vi "On Drop.vi"(8 "error in (no error)":errorcluster, 10 "Actor in":refnum<class "Actor.lvclass">, 11 "Client Connection Handler Msg in":refnum<class "Server Connection Handler Msg.lvclass">) -> (0 "error out":errorcluster, 2 "Actor out":refnum<class "Actor.lvclass">, 3 "Client Connection Handler Msg out":refnum<class "Server Connection Handler Msg.lvclass">)   [LabVIEW 2021, in "Echo Reply Test With Server Manager.lvlib" / "Server Connection Handler Msg.lvclass"]
uses:
  Server Connection Handler Msg.lvclass
  <vilib>/ActorFramework/Actor/Actor.lvclass
  Server Connection Handler Msg.lvclass/Server Connection Handler Msg.ctl
  WS Test Server Subscriber/WS Test Server Subscriber.lvclass
  C:/Program Files/National Instruments/LabVIEW 2021/vi.lib/ActorFramework/Actor/Actor.lvclass
  C:/Projects/WebSocket-Actor/Examples/Echo Reply Test With Server Manager/WS Test Server Subscriber/WS Test Server Subscriber.lvclass
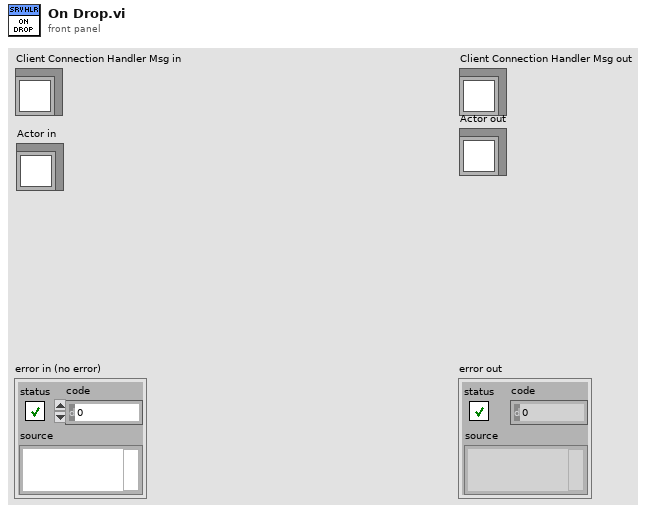
[diagram p1: front panel]
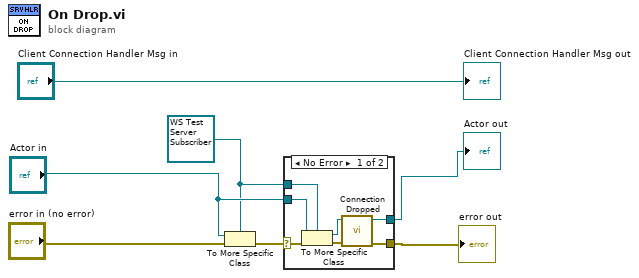
[diagram p0: block diagram]
diagram:
  w2 = refnum<class "WS Test Server Subscriber.lvclass"> refnum ("Echo Reply Test With Server Manager.lvlib:WS Test Server Subscriber.lvclass")
  n1 = To More Specific Class(target class=w2, reference="Actor in", error in="error in (no error)") -> (error out=w7:errorcluster)  [unwired: 1 out]
  n2 = case shown="No Error" w7 {
    selector: w7 -> [w13 w15]
    tunnel: [w14 w15] -> w5
    tunnel: w2 -> [w11 w16]
    tunnel: "Actor in" -> [w10 _]
    tunnel: [w8 w16] -> w3
    frame No Error {
      n3 = To More Specific Class(target class=w11, reference=w10, error in=w13) -> (specific class reference=w9:refnum<class "WS Test Server Subscriber.lvclass">, error out=w12:errorcluster)
      n4 = call "Connection Dropped.vi"("error in (no error)"=w12, "WS Test Server Subscriber in"=w9) -> ("error out"=w14:errorcluster, "WS Test Server Subscriber out"=w8:refnum<class "WS Test Server Subscriber.lvclass">)  [unwired: 8 in]
    }
    frame Error {
    }
  }
  "error out" <- w5
  "Actor out" <- w3
  "Client Connection Handler Msg out" <- "Client Connection Handler Msg in"
